vi "RealIO.vi"(10 "AllControls Out":T1) -> ()   [LabVIEW 2017]
uses:
  Ctrls/AllControls.ctl
  Ctrls/AlarmIndex.ctl
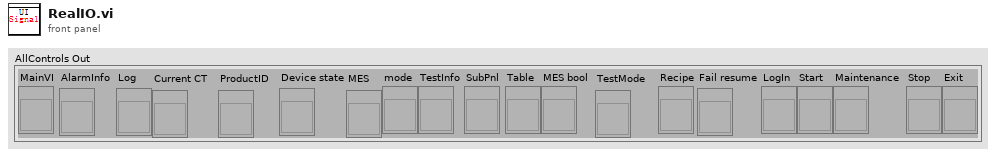
[diagram p1: front panel]
types:
  T1 = typedef "AllControls.ctl" = cluster{"MainVI":refnum<vi>, "AlarmInfo":refnum<vi>, "Log":refnum<vi>, "Current CT":refnum<vi>, "ProductID":refnum<vi>, "Device state":refnum<vi>, "MES":refnum<vi>, "mode":refnum<vi>, "TestInfo":refnum<vi>, "SubPnl":refnum<vi>, "Table":refnum<vi>, "MES bool":refnum<vi>, "TestMode":refnum<vi>, "Recipe":refnum<vi>, "Fail resume":refnum<vi>, "LogIn":refnum<vi>, "Start":refnum<vi>, "Maintenance":refnum<vi>, "Stop":refnum<vi>, "Exit":refnum<vi>}
  T2 = typedef "AlarmIndex.ctl" = enum16{"E-Stop", "Safety light grid", "UUT Sealing Cylinder HomePoint", "UUT Sealing Cylinder WorkPoint", "Orifice fixed Cylinder L HomePoint", "Orifice fixed Cylinder L WorkPoint", "Orifice fixed Cylinder R HomePoint", "Orifice fixed Cylinder R WorkPoint", "UUT Cylinder HomePoint", "UUT Cylinder WorkPoint", "Carrier fixed Cylinder L HomePoint", "Carrier fixed Cylinder L WorkPoint", "Carrier fixed Cylinder R HomePoint", "Carrier fixed Cylinder R WorkPoint", "Probe Cylinder HomePoint", "Probe Cylinder WorkPoint", "Motor Error", "Test Error"}
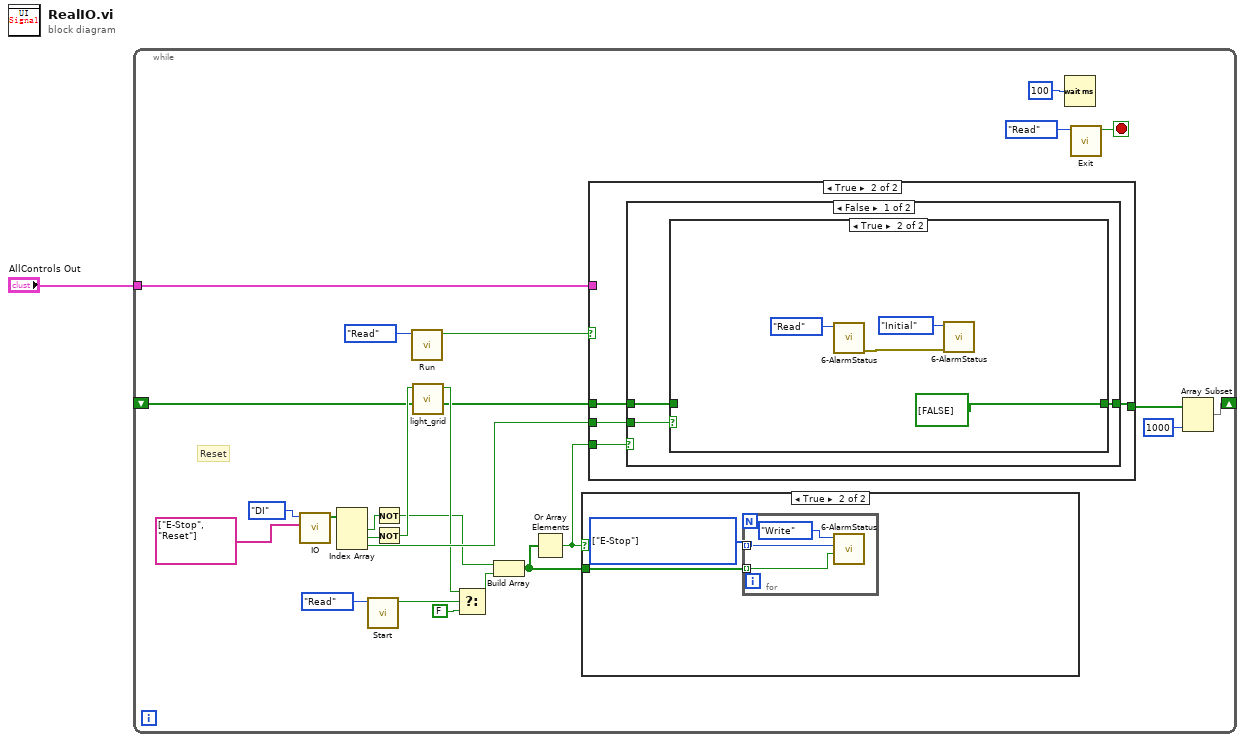
[diagram p0: block diagram]
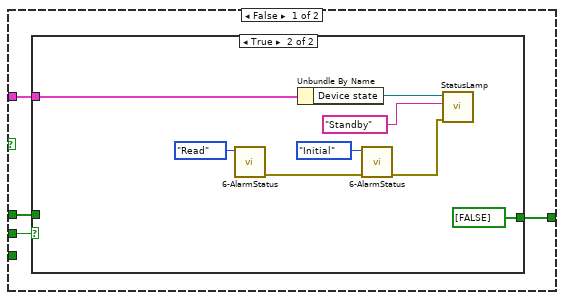
[diagram p3: hidden frame]
diagram:
  n1 = while {
    tunnel: "AllControls Out" -> [w12]
    shift-right: [w5] -> _
    shift-left: _ -> [w7]
    stop <- w27 stop-if-true
    # "Reset"
    n2 = call "IO.vi"("IO Name"=string[] ["E-Stop", "Reset"], "IO?"=enum16{"DI", "DO"}."DI") -> ("DI"=w17:bool[])  [unwired: 8 in, 1 out]
    n3 = Index Array(array=w17) -> (element #1=w22:bool, element #2=w18:bool, element #3=w16:bool)  [unwired: 3 in]
    n4 = call "Start.vi"("Step"=enum16{"Initial", "Write", "Read"}."Read") -> ("Start Out"=w20:bool)  [unwired: 9 in, 1 out]
    n5 = Not(x=w22) -> (.not. x?=w3:bool)
    n6 = Not(x=w18) -> (.not. x?=w10:bool)
    n7 = call "Run.vi"("Step"=enum16{"Initial", "Write", "Read"}."Read") -> ("Run Out"=w13:bool)  [unwired: 9 in, 1 out]
    n8 = call "light_grid.vi"("Array"=w7, "Boolean"=w10) -> ("Array 2"=w8:bool[], "logical AND"=w9:bool)  [unwired: 8 in]
    n9 = Select(t=w9, s=w20, f=FALSE) -> (s? t:f=w15:bool)
    n10 = Build Array(w3, w15) -> (w2:bool[])
    n11 = Or Array Elements(Boolean array=w2) -> (logical OR=w11:bool)
    n12 = case shown="True" w11 {
      tunnel: w2 -> [_ w28]
      frame False {
      }
      frame True {
        w29 = T2[] [enum."E-Stop"] items=["E-Stop", "Safety light grid", "UUT Sealing Cylinder HomePoint", "UUT Sealing Cylinder WorkPoint", "Orifice fixed Cylinder L HomePoint", "Orifice fixed Cylinder L WorkPoint", "Orifice fixed Cylinder R HomePoint", "Orifice fixed Cylinder R WorkPoint", "UUT Cylinder HomePoint", "UUT Cylinder WorkPoint", "Carrier fixed Cylinder L HomePoint", "Carrier fixed Cylinder L WorkPoint", "Carrier fixed Cylinder R HomePoint", "Carrier fixed Cylinder R WorkPoint", "Probe Cylinder HomePoint", "Probe Cylinder WorkPoint", "Motor Error", "Test Error"]
        n13 = for {
          tunnel: w29 -> [w32] mode=indexing
          tunnel: w28 -> [w30] mode=indexing
          n14 = call "6-AlarmStatus.vi"("AlarmValue"=w30, "AlarmIndex"=w32, "Step"=enum16{"Initial", "Write", "Read"}."Write") -> ()  [unwired: 7 in, 2 out]
        }
      }
    }
    n15 = case shown="True" w13 {
      tunnel: w16 -> [w36 w48]
      tunnel: w12 -> [w35 _]
      tunnel: w11 -> [_ w49]
      tunnel: w8 -> [w34 w46]
      tunnel: [w33 w47] -> w6
      frame False {
        n16 = case shown="True" w36 {
          tunnel: w35 -> [_ w44]
          tunnel: w34 -> [w37 _]
          tunnel: [w37 bool[] [FALSE] ("Array 2")] -> w33
          frame False {
          }
          frame True {
            n17 = call "6-AlarmStatus.vi"("Step"=enum16{"Initial", "Write", "Read"}."Read") -> ("error out"=w38:errorcluster)  [unwired: 9 in, 1 out]
            n18 = Unbundle By Name(w44) -> ("Device state"=w45:refnum<vi>)
            n19 = call "6-AlarmStatus.vi"("error in (no error)"=w38, "Step"=enum16{"Initial", "Write", "Read"}."Initial") -> ("error out"=w40:errorcluster)  [unwired: 8 in, 1 out]
            n20 = call "StatusLamp.vi"("错误输入（无错误）"=w40, "State"="Standby", "Boolean输入"=w45) -> ()  [unwired: 8 in, 1 out]
          }
        }
      }
      frame True {
        n21 = case shown="False" w49 {
          tunnel: w48 -> [w52 _]
          tunnel: [w51 w58] -> w47
          tunnel: w46 -> [w50 w58]
          frame False {
            n22 = case shown="True" w52 {
              tunnel: [w53 bool[] [FALSE] ("Array 2")] -> w51
              tunnel: w50 -> [w53 _]
              frame False {
              }
              frame True {
                n23 = call "6-AlarmStatus.vi"("Step"=enum16{"Initial", "Write", "Read"}."Read") -> ("error out"=w54:errorcluster)  [unwired: 9 in, 1 out]
                n24 = call "6-AlarmStatus.vi"("error in (no error)"=w54, "Step"=enum16{"Initial", "Write", "Read"}."Initial") -> ()  [unwired: 8 in, 2 out]
              }
            }
          }
          frame True {
          }
        }
      }
    }
    n25 = Wait (ms)(milliseconds to wait=u32 100 ("等待时间（毫秒）")) -> ()  [unwired: 1 out]
    n26 = call "Exit.vi"("Step"=enum16{"Initial", "Write", "Read"}."Read") -> ("Exit Out"=w27:bool)  [unwired: 9 in, 1 out]
    n27 = Array Subset(array=w6, length=1000) -> (w5:bool[])  [unwired: 1 in]
  }
